vi "Intersection.vi"(10 "Line2":T1, 11 "Line1":T1) -> (1 "Px":dbl, 2 "Py":dbl, 3 "denom":dbl)   [LabVIEW 2021]
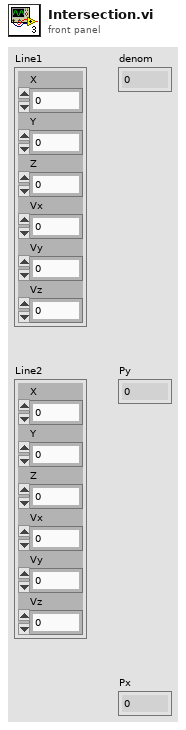
[diagram p1: front panel]
types:
  T1 = cluster{"X":ext, "Y":ext, "Z":ext, "Vx":ext, "Vy":ext, "Vz":ext}
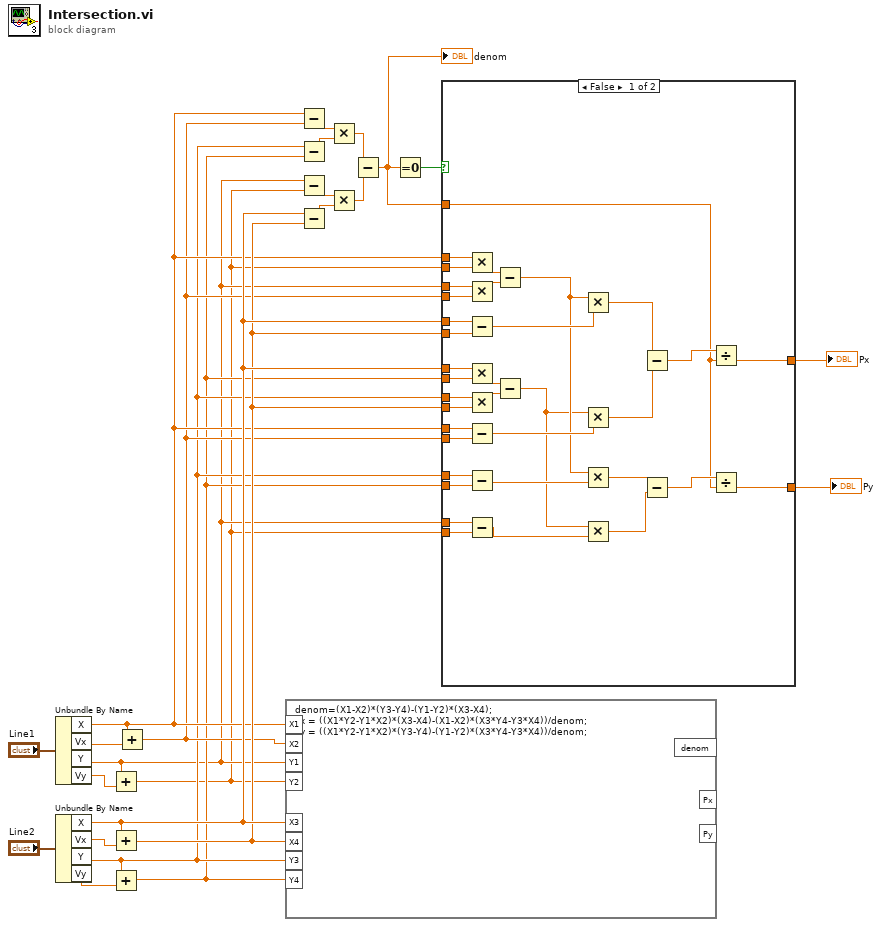
[diagram p0: block diagram]
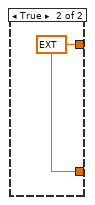
[diagram p2: hidden frame]
diagram:
  n1 = Unbundle By Name("Line1") -> ("X"=w9:ext, "Vx"=w19:ext, "Y"=w2:ext, "Vy"=w20:ext)
  n2 = Unbundle By Name("Line2") -> ("X"=w11:ext, "Vx"=w21:ext, "Y"=w4:ext, "Vy"=w22:ext)
  n3 = Add(x=w2, y=w20) -> (x+y=w1:ext)
  n4 = Add(x=w11, y=w21) -> (x+y=w10:ext)
  n5 = Add(x=w4, y=w22) -> (x+y=w3:ext)
  n6 = Add(x=w9, y=w19) -> (x+y=w8:ext)
  n7 = formula code="denom=(X1-X2)*(Y3-Y4)-(Y1-Y2)*(X3-X4);\nPx = ((X1*Y2-Y1*X2)*(X3-X4)-(X1-X2)*(X3*Y4-Y3*X4))/denom;\nPy = ((X1*Y2-Y1*X2)*(Y3-Y4)-(Y1-Y2)*(X3*Y4-Y3*X4))/denom;"("X1"=w9, "X2"=w8, "Y1"=w2, "Y2"=w1, "X3"=w11, "X4"=w10, "Y3"=w4, "Y4"=w3) -> ()  [unwired: 3 out]
  n8 = Subtract(x=w9, y=w8) -> (x-y=w18:ext)
  n9 = Subtract(x=w4, y=w3) -> (x-y=w15:ext)
  n10 = Subtract(x=w2, y=w1) -> (x-y=w16:ext)
  n11 = Subtract(x=w11, y=w10) -> (x-y=w17:ext)
  n12 = Multiply(x=w18, y=w15) -> (x*y=w13:ext)
  n13 = Multiply(x=w16, y=w17) -> (x*y=w14:ext)
  n14 = Subtract(x=w13, y=w14) -> (x-y=w5:ext)
  "denom" <- w5
  n15 = Equal To 0?(x=w5) -> (x = 0?=w12:bool)
  n16 = case shown="False" w12 {
    tunnel: w9 -> [w59 _]
    tunnel: w1 -> [w58 _]
    tunnel: w8 -> [w56 _]
    tunnel: w2 -> [w55 _]
    tunnel: w11 -> [w50 _]
    tunnel: w3 -> [w51 _]
    tunnel: w10 -> [w53 _]
    tunnel: w4 -> [w54 _]
    tunnel: w11 -> [w47 _]
    tunnel: w10 -> [w46 _]
    tunnel: w9 -> [w45 _]
    tunnel: w8 -> [w44 _]
    tunnel: [w31 w60] -> w7
    tunnel: [w30 w60] -> w6
    tunnel: w5 -> [w29 _]
    tunnel: w4 -> [w28 _]
    tunnel: w3 -> [w27 _]
    tunnel: w2 -> [w26 _]
    tunnel: w1 -> [w25 _]
    frame False {
      n17 = Multiply(x=w59, y=w58) -> (x*y=w57:ext)
      n18 = Multiply(x=w55, y=w56) -> (x*y=w49:ext)
      n19 = Subtract(x=w47, y=w46) -> (x-y=w43:ext)
      n20 = Multiply(x=w50, y=w51) -> (x*y=w52:ext)
      n21 = Multiply(x=w54, y=w53) -> (x*y=w48:ext)
      n22 = Subtract(x=w45, y=w44) -> (x-y=w42:ext)
      n23 = Subtract(x=w28, y=w27) -> (x-y=w36:ext)
      n24 = Subtract(x=w26, y=w25) -> (x-y=w33:ext)
      n25 = Subtract(x=w57, y=w49) -> (x-y=w35:ext)
      n26 = Subtract(x=w52, y=w48) -> (x-y=w34:ext)
      n27 = Multiply(x=w35, y=w43) -> (x*y=w40:ext)
      n28 = Multiply(x=w34, y=w42) -> (x*y=w41:ext)
      n29 = Multiply(x=w35, y=w36) -> (x*y=w38:ext)
      n30 = Multiply(x=w34, y=w33) -> (x*y=w37:ext)
      n31 = Subtract(x=w40, y=w41) -> (x-y=w39:ext)
      n32 = Subtract(x=w38, y=w37) -> (x-y=w32:ext)
      n33 = Divide(x=w39, y=w29) -> (x/y=w31:ext)
      n34 = Divide(x=w32, y=w29) -> (x/y=w30:ext)
    }
    frame True {
      w60 = ext nan
    }
  }
  "Py" <- w6
  "Px" <- w7
